vi "REQ full lifecycle v3.vi"(0 "endpoint":string="tcp://127.0.0.1:5555", 1 "Julia ZMQ server file name":string="ZMQ-testserver2.jl", 2 "LV Client state in":T1, 5 "data to send":string="hello", 9 "Force command":bool, 11 "error in":errorcluster, 12 "command":T2, 13 "Jl Server state in":T1) -> (3 "LV Client state out":T1, 6 "server response":string, 14 "Jl Server state out":T1, 15 "error out":errorcluster)   [LabVIEW 2018, in "LV-Julia_ZMQ-Roundtrip_lib.lvlib"]
uses:
  Commands v2.ctl
  Server or client state.ctl
  <vilib>/addons/zeromq/zmq_socket.lvclass
  <vilib>/addons/zeromq/zmq_context.lvclass
  <vilib>/Utility/error.llb/Error Cluster From Error Code.vi
  <vilib>/ErrorRing/Error Ring.xnode
  LV-Julia_ZMQ-Roundtrip_lib.lvlib
panel:
  out "return code":i32
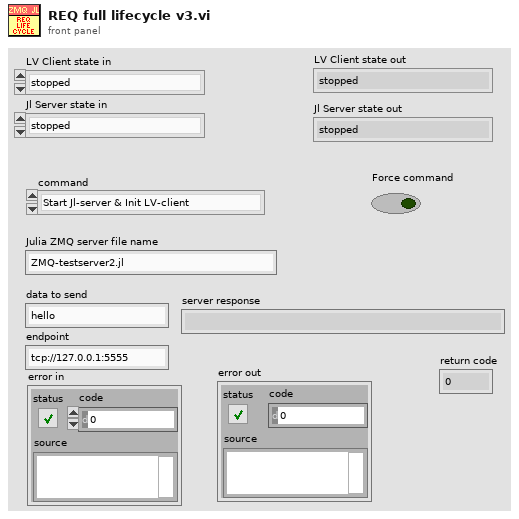
[diagram p1: front panel]
types:
  T1 = typedef "LV-Julia_ZMQ-Roundtrip_lib.lvlib/Server or client state.ctl" = enum16{"stopped", "running", "unknown"}
  T2 = typedef "LV-Julia_ZMQ-Roundtrip_lib.lvlib/Commands v2.ctl" = enum16{"Start Jl-server & Init LV-client", "Send request & Get response ", "Stop Jl-server & Cleanup LV-client", "Cleanup LV-client", "Start Jl-server", "Stop Jl-server", "Init LV-Client", "Cleanup LV-Client", "(not allowed)", "Set LV Client state", "Set Jl Server state"}
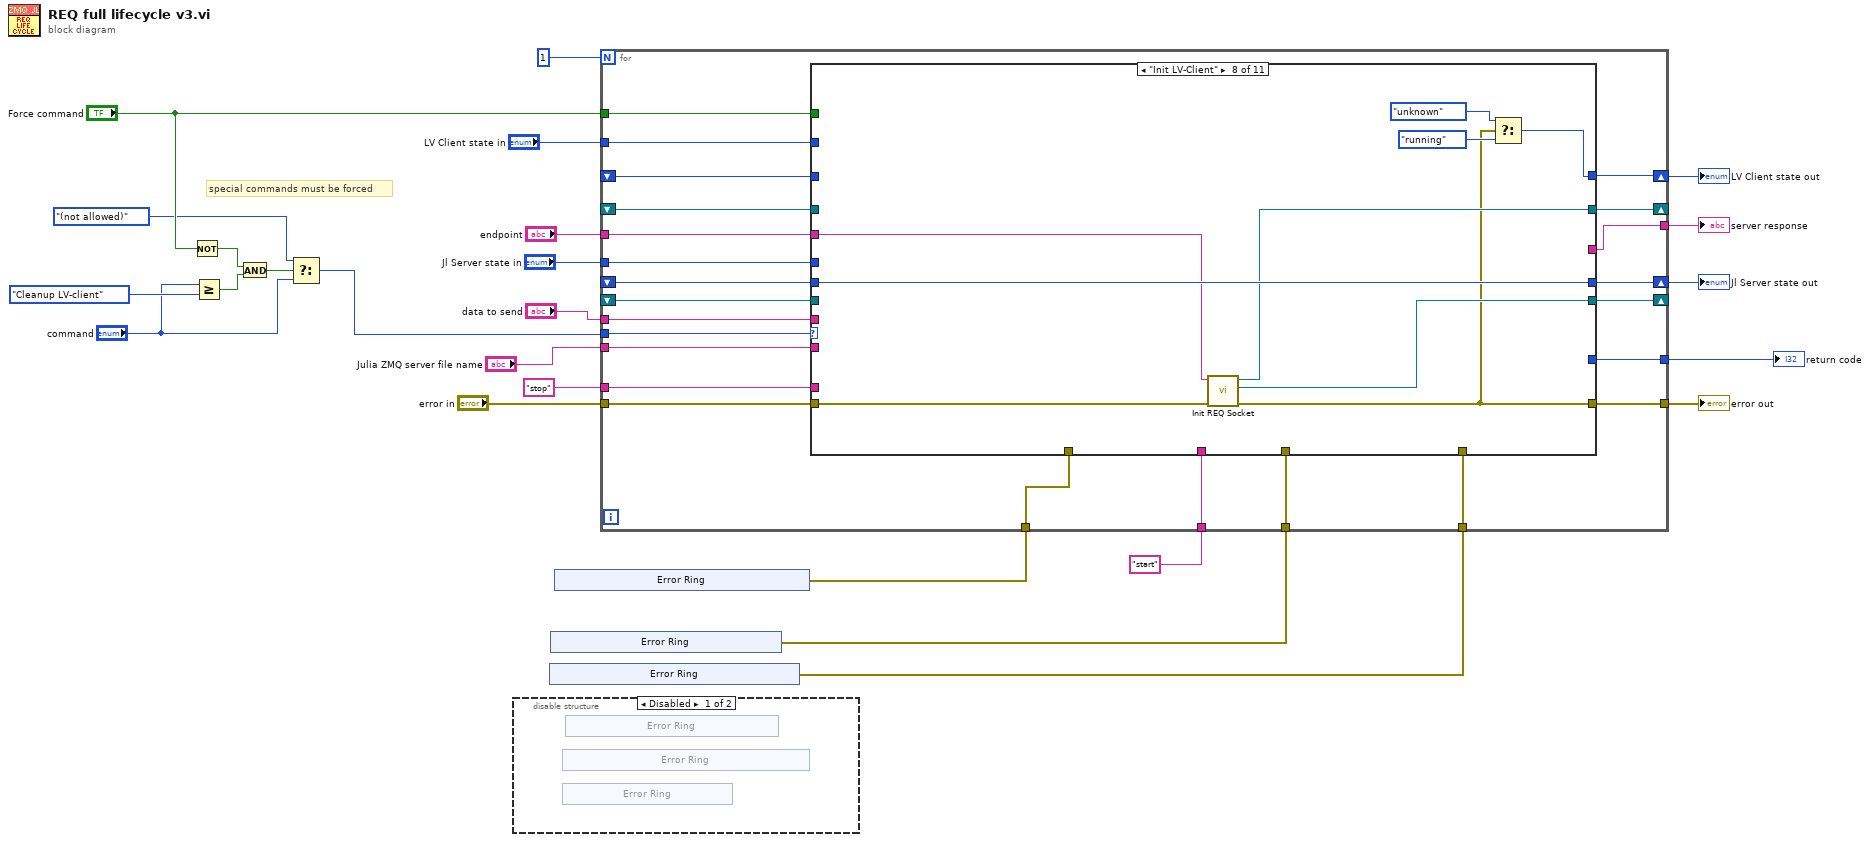
[diagram p0: block diagram]
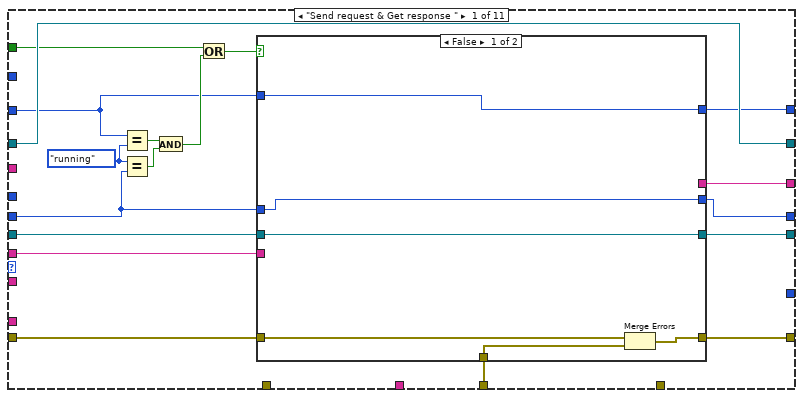
[diagram p3: hidden frame]
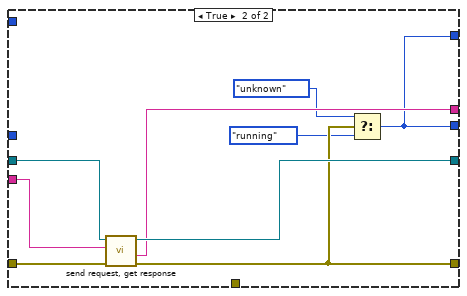
[diagram p4: hidden frame]
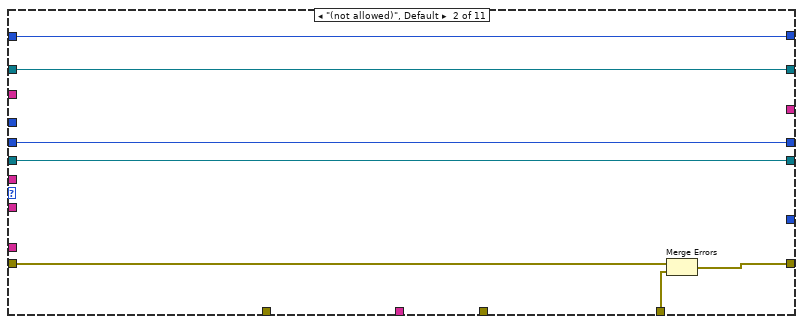
[diagram p5: hidden frame]
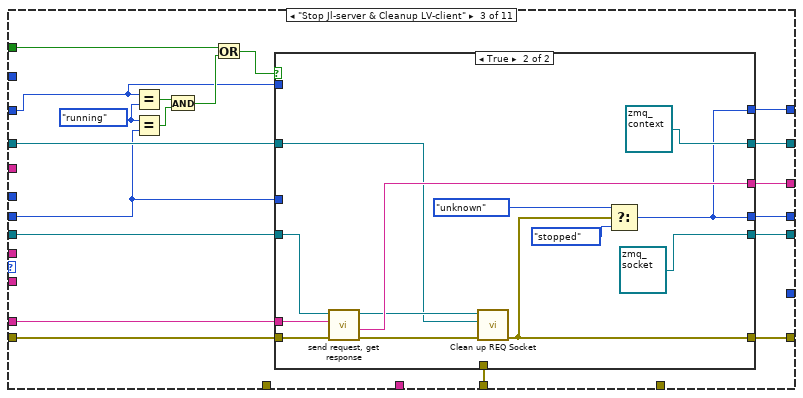
[diagram p6: hidden frame]
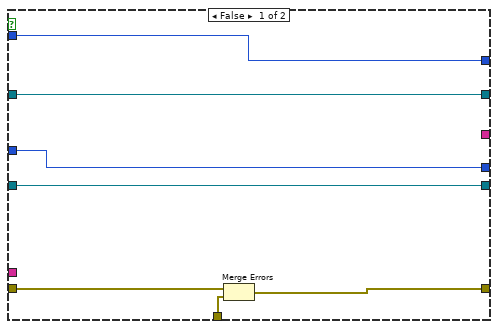
[diagram p7: hidden frame]
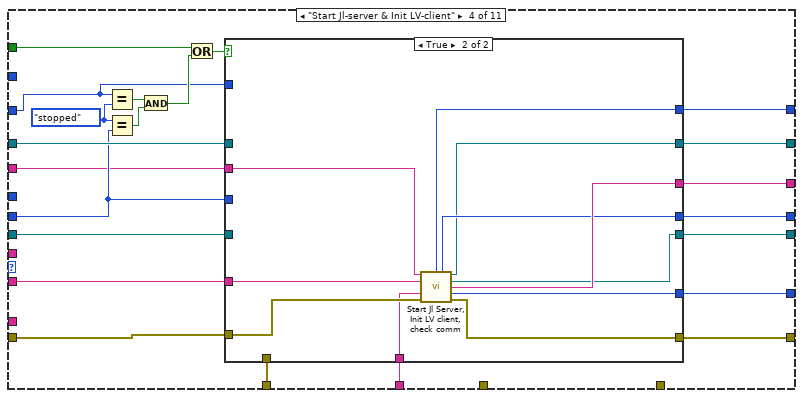
[diagram p8: hidden frame]
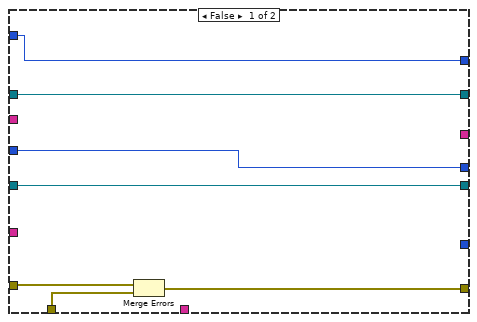
[diagram p9: hidden frame]
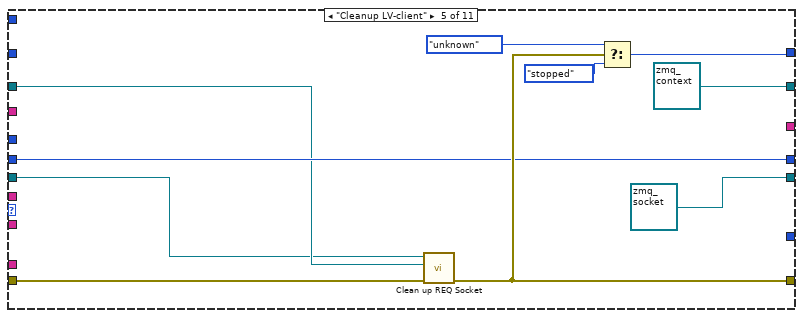
[diagram p10: hidden frame]
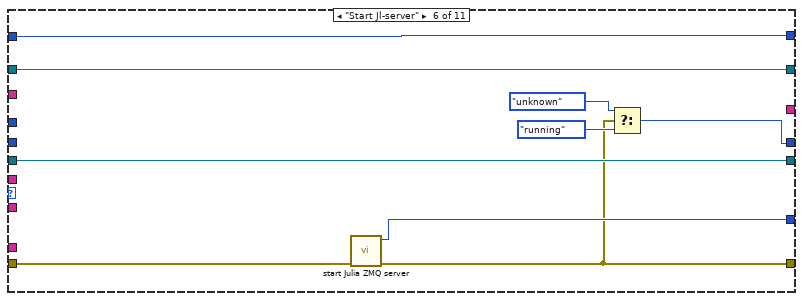
[diagram p11: hidden frame]
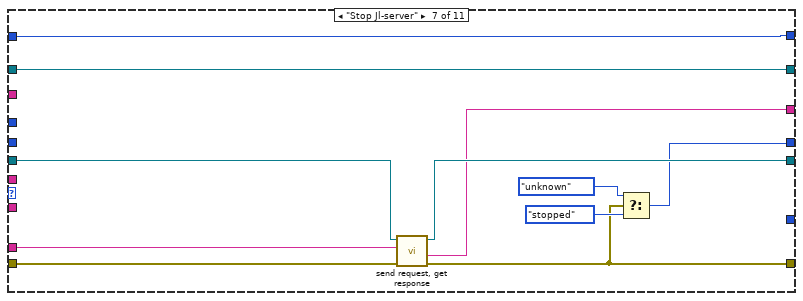
[diagram p12: hidden frame]
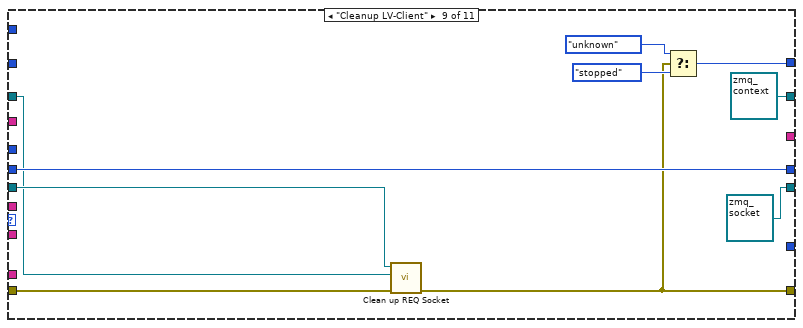
[diagram p13: hidden frame]
diagram:
  # "special commands must be forced"
  n1 = Not(x="Force command") -> (.not. x?=w10:bool)
  n2 = Greater Or Equal?(x="command", y=Commands_v2."Cleanup LV-client" ("command")) -> (x >= y?=w11:bool)
  n3 = And(x=w10, y=w11) -> (x .and. y?=w9:bool)
  n4 = Select(t=Commands_v2."(not allowed)" ("command"), s=w9, f="command") -> (s? t:f=w6:T2)
  n5 = disable-structure shown="Disabled" {
    frame Disabled {
      n6 = xnode "Error Ring"() -> ()  [unwired: 1 out]
      n7 = xnode "Error Ring"() -> ()  [unwired: 1 out]
      n8 = xnode "Error Ring"() -> ()  [unwired: 1 out]
    }
    frame Enabled {
    }
  }
  n9 = xnode "Error Ring"() -> ("error out"=w5:errorcluster)
  n10 = xnode "Error Ring"() -> ("error out"=w14:errorcluster)
  n11 = xnode "Error Ring"() -> ("error out"=w17:errorcluster)
  n12 = for {
    N: 1 -> [_]
    tunnel: [w64] -> w24
    tunnel: [w63] -> w23
    shift-right: [w62] -> _
    shift-left: _ -> [w55]
    tunnel: "endpoint" -> [w61]
    tunnel: "data to send" -> [w60]
    shift-right: [w59] -> _
    shift-left: _ -> [w54]
    tunnel: "error in" -> [w58]
    shift-right: [w56] -> w15
    shift-left: _ -> [w57]
    tunnel: w6 -> [w53]
    tunnel: "Julia ZMQ server file name" -> [w52]
    tunnel: "stop" ("request") -> [w51]
    tunnel: w17 -> [w50]
    tunnel: "start" ("request") -> [w48]
    tunnel: "Force command" -> [w49]
    shift-right: [w47] -> w4
    shift-left: _ -> [w46]
    tunnel: w14 -> [w45]
    tunnel: w5 -> [w44]
    tunnel: [w43] -> w3
    tunnel: "LV Client state in" -> [w42]
    tunnel: "Jl Server state in" -> [w41]
    n13 = case shown="\"Init LV-Client\"" w53 {
      tunnel: [w76 w103 w118 w164 w190 w194 w204 w215 w223 w234 w239] -> w64
      tunnel: [w77 _ w121 w152 _ _ w207 _ _ _ _] -> w63
      tunnel: [w82 w100 w115 w161 refnum<class "zmq_context.lvclass"> refnum ("zmq_context out") w199 w209 w217 refnum<class "zmq_context.lvclass"> refnum ("zmq_context out") w237 w241] -> w62
      tunnel: w61 -> [_ _ _ w151 _ _ _ w214 _ _ _]
      tunnel: w60 -> [w78 _ _ _ _ _ _ _ _ _ _]
      tunnel: [w80 w98 w116 w157 refnum<class "zmq_socket.lvclass"> refnum ("zmq_socket out") w198 w208 w216 refnum<class "zmq_socket.lvclass"> refnum ("socket out") w235 w240] -> w59
      tunnel: w58 -> [w81 w104 w123 w165 w193 w201 w211 w218 w226 w234 w239]
      tunnel: [w75 w99 w120 w160 w188 w195 w203 w220 w227 w236 w238] -> w56
      tunnel: w52 -> [_ _ _ w159 _ _ _ _ _ _ _]
      tunnel: w54 -> [w79 w98 w122 w158 w186 w198 w213 _ w225 w235 w240]
      tunnel: w55 -> [w82 w100 w117 w162 w187 w199 w209 _ w224 w237 w241]
      tunnel: w57 -> [w66 w99 w108 w156 w188 _ _ w220 w227 w236 _]
      tunnel: w51 -> [_ _ w119 _ _ _ w212 _ _ _ _]
      tunnel: w50 -> [_ _ _ w163 _ _ _ _ _ _ _]
      tunnel: w49 -> [w69 _ w109 w154 _ _ _ _ _ _ _]
      tunnel: w48 -> [_ _ _ w153 _ _ _ _ _ _ _]
      tunnel: [w74 w101 w107 w150 w189 w202 w210 w219 w230 w233 w242] -> w47
      tunnel: w46 -> [w67 w101 w105 w145 _ w202 w210 _ _ _ w242]
      tunnel: w45 -> [w65 _ w106 _ _ _ _ _ _ _ _]
      tunnel: w44 -> [_ w102 _ _ _ _ _ _ _ _ _]
      tunnel: [_ _ _ w144 _ w200 _ _ _ _ _] -> w43
      tunnel: w42 -> [_ _ _ _ _ _ _ _ _ w233 _]
      tunnel: w41 -> [_ _ _ _ _ _ _ _ _ _ w238]
      frame "Send request & Get response " {
        w72 = Server_or_client_state."running" ("Server state")
        n14 = Equal?(x=w67, y=w72) -> (x = y?=w70:bool)
        n15 = Equal?(x=w72, y=w66) -> (x = y?=w73:bool)
        n16 = And(x=w70, y=w73) -> (x .and. y?=w71:bool)
        n17 = Or(x=w69, y=w71) -> (x .or. y?=w68:bool)
        n18 = case shown="False" w68 {
          tunnel: w81 -> [w85 w97]
          tunnel: [w86 w96] -> w80
          tunnel: w79 -> [w86 w95]
          tunnel: w78 -> [_ w94]
          tunnel: [_ w93] -> w77
          tunnel: [w84 w91] -> w76
          tunnel: [w87 w90] -> w75
          tunnel: w66 -> [w87 _]
          tunnel: [w88 w90] -> w74
          tunnel: w67 -> [w88 _]
          tunnel: w65 -> [w83 _]
          frame False {
            n19 = Merge Errors(w85, w83) -> (w84:errorcluster)
          }
          frame True {
            n20 = call "send request, get response.vi"("error in (no error)"=w97, "request"=w94, "zmq_socket in"=w95) -> ("error out"=w91:errorcluster, "response"=w93:string, "zmq_socket out"=w96:refnum<class "zmq_socket.lvclass">)  [unwired: 4 in, 2 out]
            n21 = Select(t=Server_or_client_state."unknown" ("Server state"), s=w91, f=Server_or_client_state."running" ("Server state")) -> (s? t:f=w90:T1)
          }
        }
      }
      frame "(not allowed)", Default {
        n22 = Merge Errors(w104, w102) -> (w103:errorcluster)
      }
      frame "Stop Jl-server & Cleanup LV-client" {
        w113 = Server_or_client_state."running" ("Server state")
        n23 = Equal?(x=w105, y=w113) -> (x = y?=w111:bool)
        n24 = Equal?(x=w113, y=w108) -> (x = y?=w114:bool)
        n25 = And(x=w111, y=w114) -> (x .and. y?=w112:bool)
        n26 = Or(x=w109, y=w112) -> (x .or. y?=w110:bool)
        n27 = case shown="True" w110 {
          tunnel: w123 -> [w126 w143]
          tunnel: w122 -> [w128 w142]
          tunnel: [_ w141] -> w121
          tunnel: [w130 w131] -> w120
          tunnel: w119 -> [_ w139]
          tunnel: [w125 w137] -> w118
          tunnel: w117 -> [w127 w134]
          tunnel: [w128 refnum<class "zmq_socket.lvclass"> refnum ("zmq_socket out")] -> w116
          tunnel: [w127 refnum<class "zmq_context.lvclass"> refnum ("zmq_context out")] -> w115
          tunnel: w108 -> [w130 _]
          tunnel: [w129 w131] -> w107
          tunnel: w105 -> [w129 _]
          tunnel: w106 -> [w124 _]
          frame False {
            n28 = Merge Errors(w126, w124) -> (w125:errorcluster)
          }
          frame True {
            n29 = call "send request, get response.vi"("error in (no error)"=w143, "request"=w139, "zmq_socket in"=w142) -> ("error out"=w138:errorcluster, "response"=w141:string, "zmq_socket out"=w135:refnum<class "zmq_socket.lvclass">)  [unwired: 4 in, 2 out]
            n30 = call "Clean up REQ Socket.vi"("error in (no error)"=w138, "zmq_context in"=w134, "zmq_socket in"=w135) -> ("error out"=w137:errorcluster)  [unwired: 8 in]
            n31 = Select(t=Server_or_client_state."unknown" ("Server state"), s=w137, f=Server_or_client_state."stopped") -> (s? t:f=w131:T1)
          }
        }
      }
      frame "Start Jl-server & Init LV-client" {
        w148 = Server_or_client_state."stopped" ("Server state")
        n32 = Equal?(x=w145, y=w148) -> (x = y?=w146:bool)
        n33 = Equal?(x=w148, y=w156) -> (x = y?=w149:bool)
        n34 = And(x=w146, y=w149) -> (x .and. y?=w147:bool)
        n35 = Or(x=w154, y=w147) -> (x .or. y?=w155:bool)
        n36 = case shown="True" w155 {
          tunnel: w165 -> [w172 w183]
          tunnel: [w171 w182] -> w164
          tunnel: w163 -> [w170 _]
          tunnel: [w169 w176] -> w161
          tunnel: w162 -> [w169 _]
          tunnel: [w168 w177] -> w160
          tunnel: w156 -> [w168 _]
          tunnel: w159 -> [_ w181]
          tunnel: [w167 w175] -> w157
          tunnel: w158 -> [w167 _]
          tunnel: w153 -> [_ w180]
          tunnel: [_ w179] -> w152
          tunnel: w151 -> [_ w178]
          tunnel: [w166 w174] -> w150
          tunnel: w145 -> [w166 _]
          tunnel: [_ w173] -> w144
          frame False {
            n37 = Merge Errors(w172, w170) -> (w171:errorcluster)
          }
          frame True {
            n38 = call "Start Jl Server, Init LV client, check comm.vi"("endpoint"=w178, "Julia ZMQ server file name"=w181, "request"=w180, "error in (no error)"=w183) -> ("LV client state"=w174:T1, "JL server state"=w177:T1, "zmq_context out"=w176:refnum<class "zmq_context.lvclass">, "zmq_socket out"=w175:refnum<class "zmq_socket.lvclass">, "response"=w179:string, "return code"=w173:i32, "error out"=w182:errorcluster)  [unwired: 5 in]
          }
        }
      }
      frame "Cleanup LV-client" {
        n39 = call "Clean up REQ Socket.vi"("error in (no error)"=w193, "zmq_context in"=w187, "zmq_socket in"=w186) -> ("error out"=w190:errorcluster)  [unwired: 8 in]
        n40 = Select(t=Server_or_client_state."unknown" ("Server state"), s=w190, f=Server_or_client_state."stopped") -> (s? t:f=w189:T1)
      }
      frame "Start Jl-server" {
        n41 = call "start Julia ZMQ server.vi"("error in (no error)"=w201) -> ("error out"=w194:errorcluster, "return code"=w200:i32)  [unwired: 9 in]
        n42 = Select(t=Server_or_client_state."unknown" ("Server state"), s=w194, f=Server_or_client_state."running") -> (s? t:f=w195:T1)
      }
      frame "Stop Jl-server" {
        n43 = call "send request, get response.vi"("error in (no error)"=w211, "request"=w212, "zmq_socket in"=w213) -> ("error out"=w204:errorcluster, "response"=w207:string, "zmq_socket out"=w208:refnum<class "zmq_socket.lvclass">)  [unwired: 4 in, 2 out]
        n44 = Select(t=Server_or_client_state."unknown" ("Server state"), s=w204, f=Server_or_client_state."stopped") -> (s? t:f=w203:T1)
      }
      frame "Init LV-Client" {
        n45 = call "Init REQ Socket.vi"("error in (no error)"=w218, "endpoint"=w214) -> ("error out"=w215:errorcluster, "socket out"=w216:refnum<class "zmq_socket.lvclass">, "zmq_context out"=w217:refnum<class "zmq_context.lvclass">)  [unwired: 7 in]
        n46 = Select(t=Server_or_client_state."unknown" ("Server state"), s=w215, f=Server_or_client_state."running") -> (s? t:f=w219:T1)
      }
      frame "Cleanup LV-Client" {
        n47 = call "Clean up REQ Socket.vi"("error in (no error)"=w226, "zmq_context in"=w224, "zmq_socket in"=w225) -> ("error out"=w223:errorcluster)  [unwired: 8 in]
        n48 = Select(t=Server_or_client_state."unknown" ("Server state"), s=w223, f=Server_or_client_state."stopped") -> (s? t:f=w230:T1)
      }
      frame "Set LV Client state" {
      }
      frame "Set Jl Server state" {
      }
    }
  }
  "error out" <- w24
  "server response" <- w23
  "Jl Server state out" <- w15
  "LV Client state out" <- w4
  "return code" <- w3
